vi "VI Tree.vi"   [LabVIEW 2021, in "Agilent 34420.lvlib"]
doc: "This is the instrument driver for the Agilent 34420. The VI Tree displays all the user-callable VIs of the instrument driver in an organized table."
uses:
  <instrlib>/Agilent 34420/Agilent 34420.lvlib
  <instrlib>/Agilent 34420/Public/Data/Read (Single Point).vi
  <instrlib>/Agilent 34420/Public/Configure/Configure Temperature (FRTD).vi
panel:
  # "(c) 2008-2015 National Instruments Corp.  ALL RIGHTS RESERVED."
  # "SEE DIAGRAM\nFOR VI TREE."
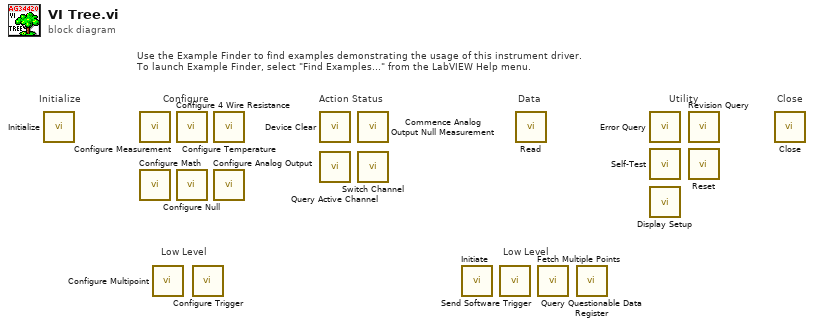
[diagram p0: block diagram]
diagram:
  # "Action Status"
  # "Low Level"
  # "Low Level"
  # "Use the Example Finder to find examples demonstrating the usage of this instrument driver.\nTo launch Example Finder, select \"Find Examples...\" from the LabVIEW Help menu."
  # "Configure"
  # "Utility"
  # "Data"
  # "Close"
  # "Initialize"
  n1 = call <instrlib>:"Initialize.vi"() -> ()  [unwired: 10 in, 2 out]
  n2 = call <instrlib>:"Configure Measurement.vi"() -> ()  [unwired: 14 in, 2 out]
  n3 = call <instrlib>:"Configure Math.vi"() -> ()  [unwired: 14 in, 2 out]
  n4 = call <instrlib>:"Configure Multipoint.vi"() -> ()  [unwired: 10 in, 2 out]
  n5 = call <instrlib>:"Configure 4 Wire Resistance.vi"() -> ()  [unwired: 14 in, 2 out]
  n6 = call <instrlib>:"Configure Null.vi"() -> ()  [unwired: 14 in, 2 out]
  n7 = call <instrlib>:"Configure Trigger.vi"() -> ()  [unwired: 14 in, 2 out]
  n8 = call-poly <instrlib>:"Configure Temperature.vi"() -> ()  [unwired: 14 in, 2 out]
  n9 = call <instrlib>:"Configure Analog Output.vi"() -> ()  [unwired: 14 in, 2 out]
  n10 = call <instrlib>:"Device Clear.vi"() -> ()  [unwired: 10 in, 2 out]
  n11 = call <instrlib>:"Query Active Channel.vi"() -> ()  [unwired: 9 in, 3 out]
  n12 = call <instrlib>:"Commence Analog Output Null Measurement.vi"() -> ()  [unwired: 10 in, 2 out]
  n13 = call <instrlib>:"Switch Channel.vi"() -> ()  [unwired: 10 in, 2 out]
  n14 = call <instrlib>:"Initiate.vi"() -> ()  [unwired: 10 in, 2 out]
  n15 = call <instrlib>:"Send Software Trigger.vi"() -> ()  [unwired: 10 in, 2 out]
  n16 = call-poly <instrlib>:"Read.vi"() -> ()  [unwired: 13 in, 3 out]
  n17 = call <instrlib>:"Fetch Multiple Points.vi"() -> ()  [unwired: 9 in, 3 out]
  n18 = call <instrlib>:"Query Questionable Data Register.vi"() -> ()  [unwired: 9 in, 3 out]
  n19 = call <instrlib>:"Error Query.vi"() -> ()  [unwired: 8 in, 4 out]
  n20 = call <instrlib>:"Self-Test.vi"() -> ()  [unwired: 8 in, 4 out]
  n21 = call <instrlib>:"Display Setup.vi"() -> ()  [unwired: 14 in, 2 out]
  n22 = call <instrlib>:"Revision Query.vi"() -> ()  [unwired: 8 in, 4 out]
  n23 = call <instrlib>:"Reset.vi"() -> ()  [unwired: 10 in, 2 out]
  n24 = call <instrlib>:"Close.vi"() -> ()  [unwired: 11 in, 1 out]
